vi "sub_calc obstacle cost.vi"   [LabVIEW 2019]
uses:
  Ctrl/cmd_common.ctl
types:
  T1 = typedef "cmd_common.ctl" = enum16{"read", "write"}
  T2 = cluster{"max speed":dbl, "min speed":dbl, "max yaw rate":dbl, "max accel":dbl, "max delta yaw rate":dbl, "v resolution":dbl, "yaw rate resolution":dbl, "dt":dbl, "predict time":dbl, "to goal cost gain":dbl, "speed cost gain":dbl, "obstacle cost gain":dbl, "robot stuck flag cons":dbl, "robot type":i8, "robot radius":dbl, "robot width":dbl, "robot length":dbl, "obstacles":cluster{"x":dbl, "y":dbl}[], "goal pt":cluster{"x":i32, "y":i32}}
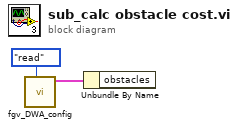
[diagram p0: block diagram]
diagram:
  n1 = call "fgv_DWA_config.vi"("cmd"=cmd_common."read") -> ("config out"=w1:T2)  [unwired: 10 in]
  n2 = Unbundle By Name(w1) -> ()  [unwired: 1 out]
